vi "testOscillation.vi"(8 "error in (no error)":errorcluster, 11 "reference in":refnum<class "subject.lvclass">) -> (0 "error out":errorcluster, 3 "reference out":refnum<class "subject.lvclass">)   [LabVIEW 2015, in "subject.lvclass"]
uses:
  subject.lvclass
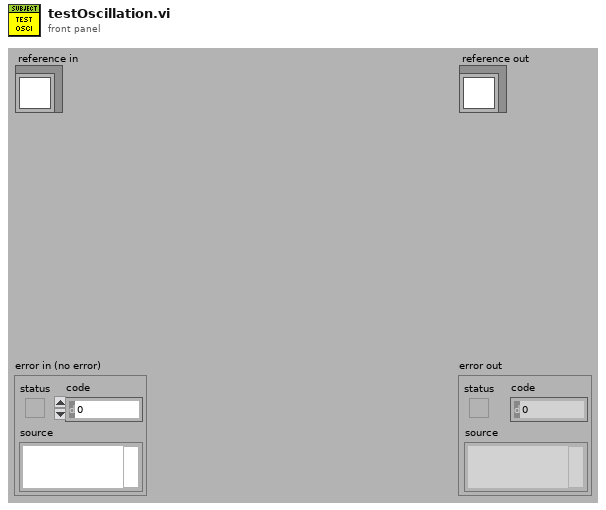
[diagram p1: front panel]
types:
  T1 = typedef "subject.lvclass/ObjectAttributesRef.ctl" = refnum<data-value>
  T2 = typedef "subject.lvclass/ObjectAttributes.ctl" = cluster{"MyAttribute":dbl, "data":cluster{"Ve_warm":dbl[], "time_warm":dbl[], "name":string, "phase":dbl[], "VCO2":dbl[], "VO2":dbl[], "PetCO2":dbl[], "RQ":dbl[], "HR":dbl[], "Ve_warm_inter":dbl[], "time_warm_inter":dbl[], "Ve_exer":dbl[], "time_exer":dbl[], "Ve_exer_inter":dbl[], "time_exer_inter":dbl[], "Ve":dbl[], "time":dbl[]}, "results_5l":cluster{"EOV":bool, "osci_amplitude":dbl[], "osci_width":dbl[], "peak_location":dbl[]}, "results_15percent":cluster{"EOV":bool, "osci_amplitude":dbl[], "osci_width":dbl[], "peak_location":dbl[]}, "supportData":cluster{"peaksAmplitude":dbl[], "iPeaksLocation":dbl[], "valesAmplitude":dbl[], "iValesLocation":dbl[], "threshold":dbl, "width_warm":i32, "meanAmpl_warm":i32, "#_peaks":i32}}
  T3 = cluster{"Ve_warm":dbl[], "time_warm":dbl[], "name":string, "phase":dbl[], "VCO2":dbl[], "VO2":dbl[], "PetCO2":dbl[], "RQ":dbl[], "HR":dbl[], "Ve_warm_inter":dbl[], "time_warm_inter":dbl[], "Ve_exer":dbl[], "time_exer":dbl[], "Ve_exer_inter":dbl[], "time_exer_inter":dbl[], "Ve":dbl[], "time":dbl[]}
  T4 = cluster{"peaksAmplitude":dbl[], "iPeaksLocation":dbl[], "valesAmplitude":dbl[], "iValesLocation":dbl[], "threshold":dbl, "width_warm":i32, "meanAmpl_warm":i32, "#_peaks":i32}
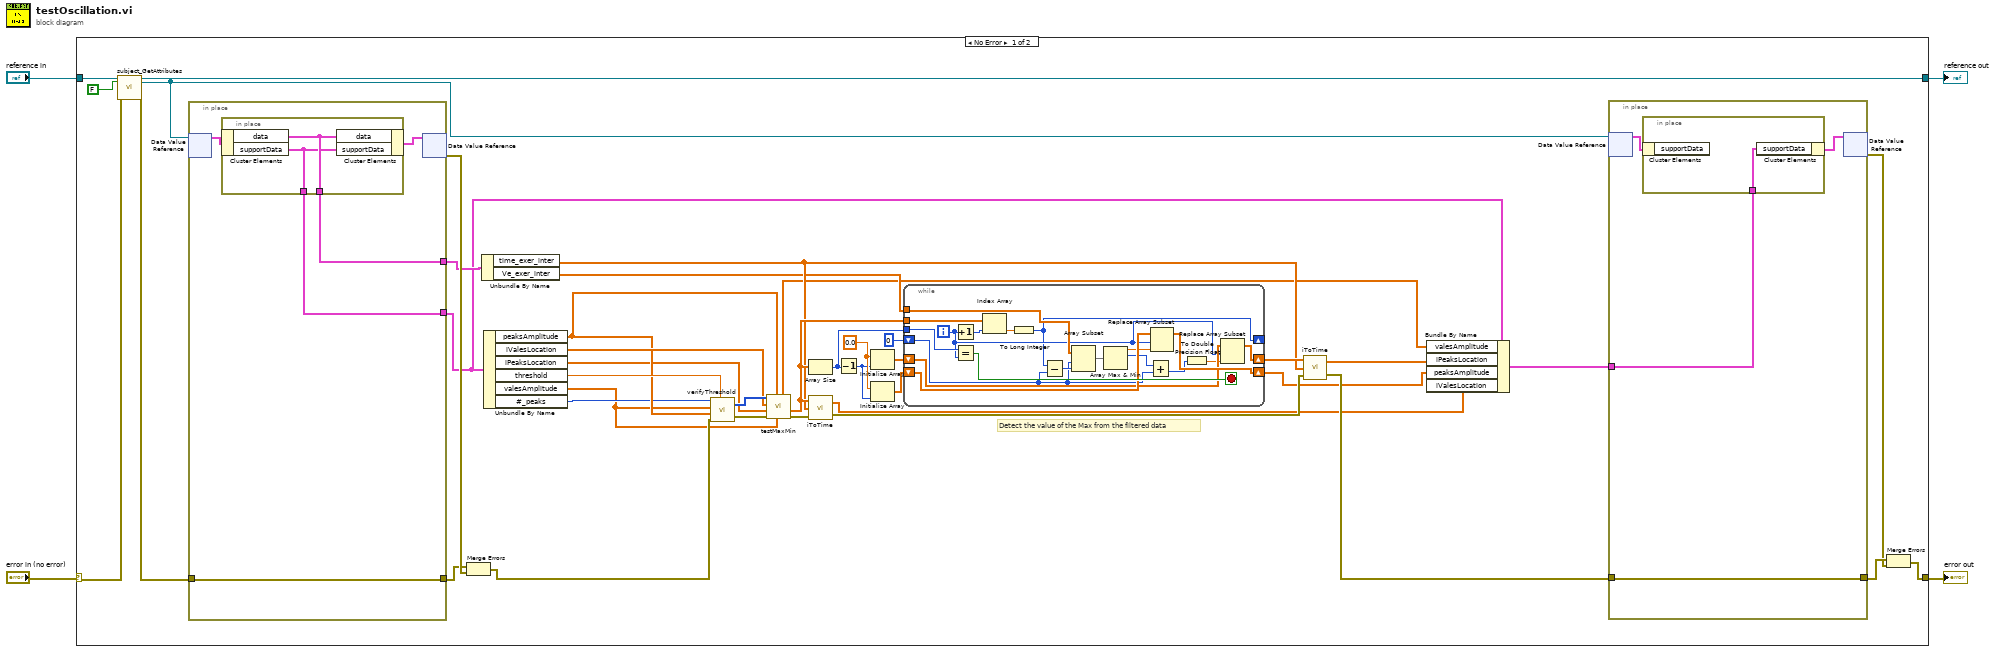
[diagram p0: block diagram]
diagram:
  n1 = case shown="No Error" "error in (no error)" {
    selector: "error in (no error)" -> [w40 w77]
    tunnel: [w13 w77] -> w3
    tunnel: [w38 w76] -> w1
    tunnel: "reference in" -> [w42 w76]
    frame No Error {
      w33 = 0.0 ("element")
      # "Detect the value of the Max from the filtered data"
      n2 = call "subject_GetAttributes.vi"("reference in"=w42, "return data? (T)"=FALSE, "error in (no error)"=w40) -> ("reference out"=w38:refnum<class "subject.lvclass">, "attributes ref"=w12:T1, "error out"=w39:errorcluster)  [unwired: 13 in, 1 out]
      n3 = in-place {
        in-place-border: w39 -> [w71]
        in-place-border: [w71] -> w43
        in-place-border: [w70] -> w11
        in-place-border: [w69] -> w10
        n4 = in-place-dvr #1(w12) -> (w72:T2)  [unwired: 1 out]
        n5 = in-place {
          in-place-border: [w75] -> w70
          in-place-border: [w74] -> w69
          n6 = in-place-cluster #2(w72) -> ("data"=w75:T3, "supportData"=w74:T4)
          n7 = in-place-cluster #2("data"=w75, "supportData"=w74) -> (w73:T2)
        }
        n8 = in-place-dvr #1(w73) -> (w44:errorcluster)  [unwired: 1 out]
      }
      n9 = Merge Errors(w43, w44) -> (w19:errorcluster)
      n10 = Unbundle By Name(w11) -> ("time_exer_inter"=w25:dbl[], "Ve_exer_inter"=w24:dbl[])
      n11 = Unbundle By Name(w10) -> ("peaksAmplitude"=w21:dbl[], "iValesLocation"=w23:dbl[], "iPeaksLocation"=w18:dbl[], "threshold"=w22:dbl, "valesAmplitude"=w17:dbl[], "#_peaks"=w20:i32)
      n12 = call "verifyThreshold.vi"("#Peaks"=w20, "valesAmplitude"=w17, "peaksAmplitude"=w21, "Error In"=w19, "threshold"=w22) -> ("passThreshold"=w37:i32[], "Error Out"=w36:errorcluster)
      n13 = call "testMaxMin.vi"("valesAmplitude in"=w17, "peaksAmplitude in"=w21, "Error In"=w36, "iPeaksLocation in"=w18, "iValesLocation in"=w23, "passThreshold"=w37) -> ("Error Out"=w30:errorcluster, "iValesLocation out"=w26:dbl[], "valesAmplitude out"=w8:dbl[])  [unwired: 2 out]
      n14 = Array Size(array=w26) -> (size(s)=w28:i32)
      n15 = call "iToTime.vi"("Error In"=w30, "time"=w25, "iArray"=w26) -> ("Error Out"=w29:errorcluster, "timeArray"=w6:dbl[])
      n16 = Decrement(x=w28) -> (x-1=w27:i32)
      n17 = Initialize Array(w33, w27) -> (w32:dbl[])
      n18 = Initialize Array(w33, w27) -> (w34:dbl[])
      n19 = while {
        tunnel: w26 -> [w68]
        tunnel: w28 -> [w67]
        tunnel: w24 -> [w64]
        shift-right: [w50] -> _
        shift-left: 0 -> [w51]
        shift-right: [w61] -> w5
        shift-left: w34 -> [w62]
        shift-right: [w59] -> w31
        shift-left: w32 -> [w60]
        i -> [w58]
        stop <- w66 stop-if-true
        n20 = Increment(x=w58) -> (x+1=w54:i32)
        n21 = Equal?(x=w67, y=w58) -> (x = y?=w66:bool)
        n22 = Index Array(array=w68, index=w54) -> (element=w65:dbl)
        n23 = To Long Integer(number=w65) -> (32bit integer=w50:i32)
        n24 = Subtract(x=w50, y=w51) -> (x-y=w52:i32)
        n25 = Array Subset(array=w64, index=w51, length=w52) -> (w63:dbl[])
        n26 = Array Max & Min(array=w63) -> (max value=w56:dbl, max index (indices)=w57:i32)  [unwired: 2 out]
        n27 = Add(x=w57, y=w51) -> (x+y=w53:i32)
        n28 = Replace Array Subset(array=w62, new element=w56, index=w58) -> (w61:dbl[])
        n29 = To Double Precision Float(number=w53) -> (double precision float=w55:dbl)
        n30 = Replace Array Subset(array=w60, new element=w55, index=w58) -> (w59:dbl[])
      }
      n31 = call "iToTime.vi"("Error In"=w29, "time"=w25, "iArray"=w31) -> ("Error Out"=w16:errorcluster, "timeArray"=w7:dbl[])
      n32 = Bundle By Name(cluster=w10, "valesAmplitude"=w8, "iPeaksLocation"=w7, "peaksAmplitude"=w5, "iValesLocation"=w6) -> (w9:T4)
      n33 = in-place {
        in-place-border: w16 -> [w46]
        in-place-border: [w46] -> w15
        in-place-border: w9 -> [w45]
        n34 = in-place-dvr #3(w12) -> (w47:T2)  [unwired: 1 out]
        n35 = in-place {
          in-place-border: w45 -> [w49]
          n36 = in-place-cluster #4(w47) -> ()  [unwired: 1 out]
          n37 = in-place-cluster #4("supportData"=w49) -> (w48:T2)
        }
        n38 = in-place-dvr #3(w48) -> (w14:errorcluster)  [unwired: 1 out]
      }
      n39 = Merge Errors(w15, w14) -> (w13:errorcluster)
    }
    frame Error {
    }
  }
  "error out" <- w3
  "reference out" <- w1
